vi "ExportDialog.vi"(0 "Int duplex ctl":refnum<vi>, 1 "16 bit ctl":refnum<vi>, 2 "coincidence image ctl":refnum<vi>, 3 "Path":refnum<vi>, 4 "notes 2":refnum<vi>) -> ()   [LabVIEW 2009]
uses:
  <vilib>/vision/Image Controls.llb/IMAQ Image.ctl
panel:
  in  "I16-File":bool
  in  "16 bit Image":bool
  in  "colorpal 16bit":T1(ring)
  in  "stop":bool
  in  "coincidence":bool
  in  "Int dup":bool
  in  "RGB/False":bool
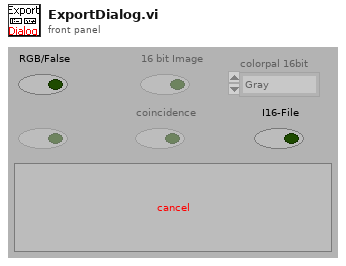
[diagram p1: front panel]
types:
  T1 = enum32{"Gray", "Binary", "Gradient", "Rainbow", "Temperature"}
  T2 = enum16{"Ini", "Get", "Set", "Refresh", "dump", "move", "name"}
  T3 = enum16{"Ini", "Dump", "Colorpal", "Input", "Get"}
  T4 = typedef "IMAQ Image.ctl" = refnum<image>
  T5 = enum16{"Get", "Set", "Change", "ini", "clear", "draw", "draw false"}
  T6 = enum16{"Ini", "Get", "Set", "Draw", "Colorpal", "Dump"}
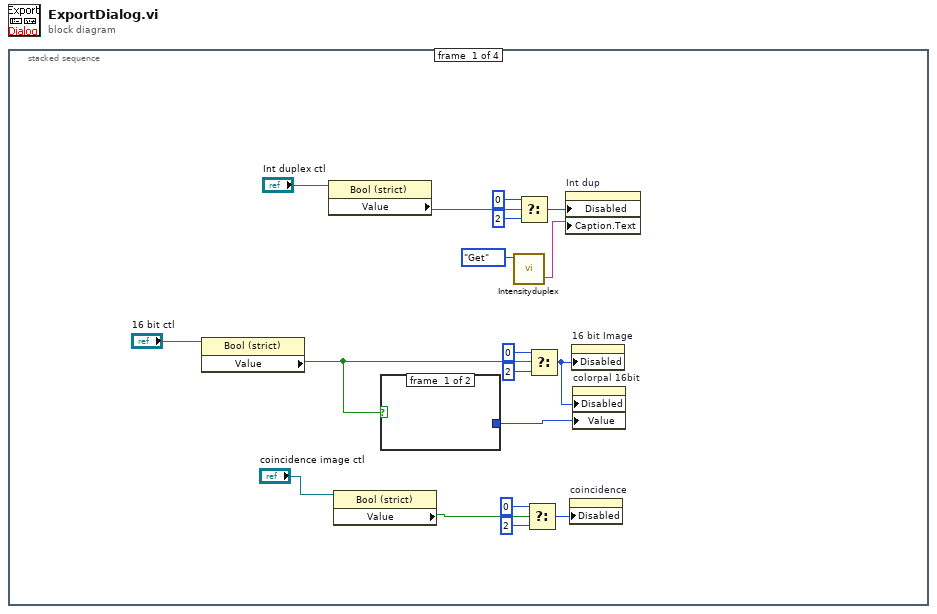
[diagram p0: block diagram]
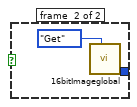
[diagram p2: hidden frame]
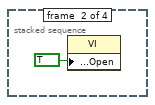
[diagram p3: hidden frame]
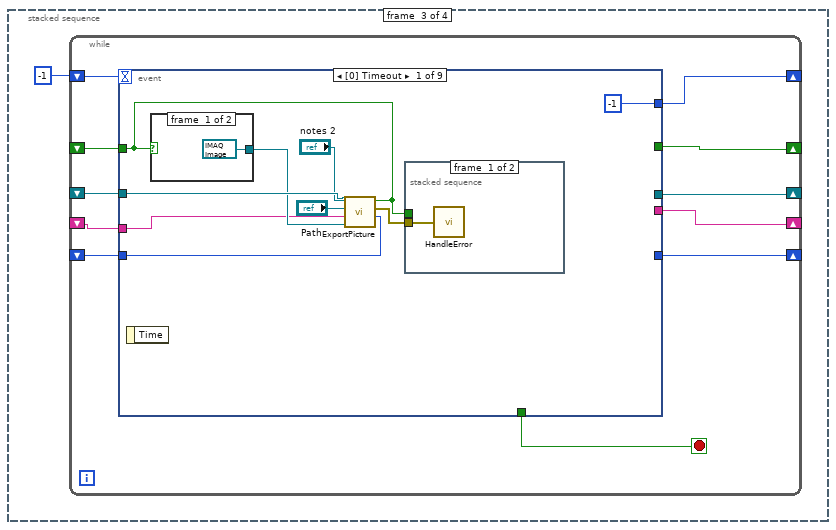
[diagram p4: hidden frame]
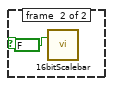
[diagram p6: hidden frame]
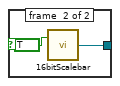
[diagram p7: hidden frame]
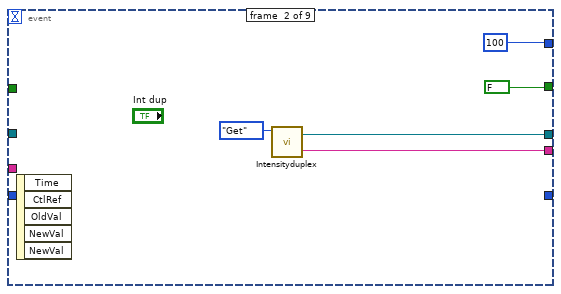
[diagram p8: hidden frame]
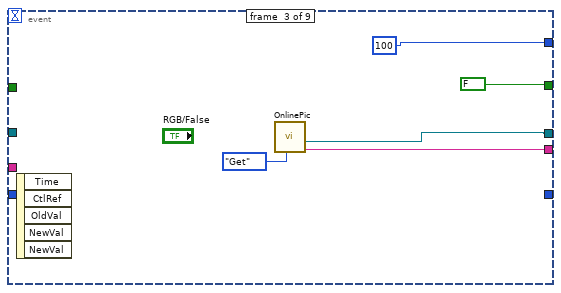
[diagram p9: hidden frame]
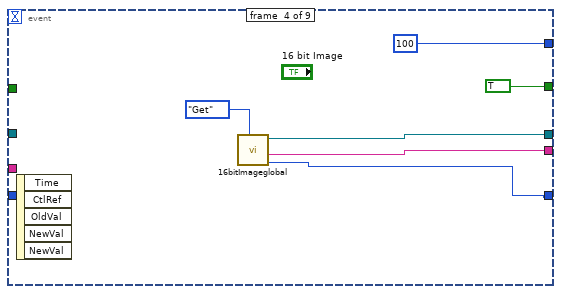
[diagram p10: hidden frame]
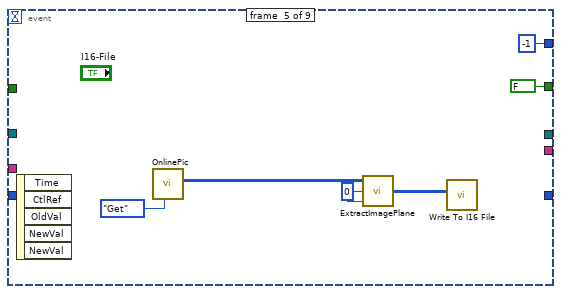
[diagram p11: hidden frame]
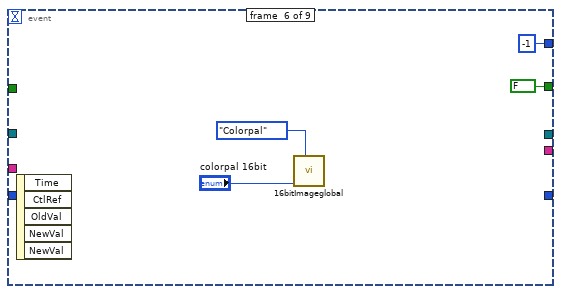
[diagram p12: hidden frame]
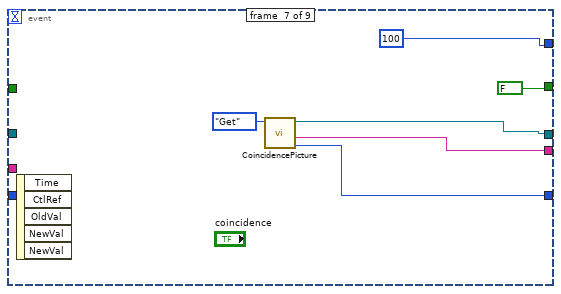
[diagram p13: hidden frame]
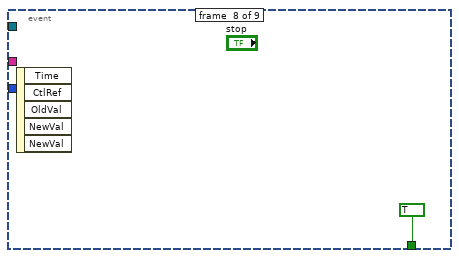
[diagram p14: hidden frame]
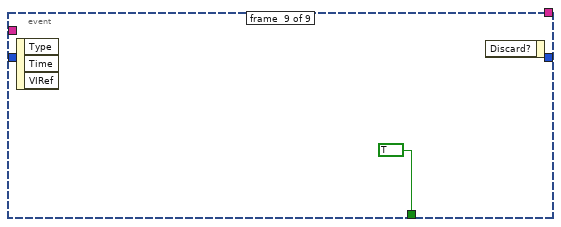
[diagram p15: hidden frame]
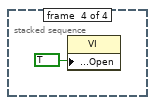
[diagram p16: hidden frame]
diagram:
  n1 = stacked-sequence {
    frame #0 {
      n2 = property on="Property Node" class="Bool (strict)"(reference="16 bit ctl") -> ("Value"=w2:bool)  [unwired: 1 in, 2 out]
      n3 = property on="Property Node" class="Bool (strict)"(reference="Int duplex ctl") -> ("Value"=w13:bool)  [unwired: 1 in, 2 out]
      n4 = property on="Property Node" class="Bool (strict)"(reference="coincidence image ctl") -> ("Value"=w9:bool)  [unwired: 1 in, 2 out]
      n5 = case shown="False" w2 {
        tunnel: [_ w19] -> w3
        frame #0 {
        }
        frame #1 {
          n6 = call "16bitImageglobal.vi"("Enum"=T3."Get") -> ("Palette Number (gray) 2"=w19:T1)  [unwired: 4 in, 3 out]
        }
      }
      n7 = call "Intensityduplex.vi"("Enum"=T2."Get") -> ("title out"=w10:string)  [unwired: 4 in, 1 out]
      n8 = Select(t=0, s=w13, f=2) -> (s? t:f=w14:i32)
      n9 = Select(t=0, s=w9, f=2) -> (s? t:f=w6:i32)
      n10 = Select(t=0, s=w2, f=2) -> (s? t:f=w4:i32)
      n11 = property on="Int dup" class="Bool"("Disabled"=w14, "Caption.Text"=w10) -> ()  [unwired: 2 in, 2 out]
      n12 = property on="coincidence" class="Bool"("Disabled"=w6) -> ()  [unwired: 2 in, 2 out]
      n13 = property on="16 bit Image" class="Bool"("Disabled"=w4) -> ()  [unwired: 2 in, 2 out]
      n14 = property on="colorpal 16bit" class="Enum (strict)"("Disabled"=w4, "Value"=w3) -> ()  [unwired: 2 in, 2 out]
    }
    frame #1 {
      n15 = property class="VI"("Front Panel Window:Open"=TRUE) -> ()  [unwired: 2 in, 2 out]
    }
    frame #2 {
      n16 = while {
        shift-right: [w31] -> _
        shift-left: -1 -> [w32]
        shift-right: [w30] -> _
        shift-left: _ -> [w25]
        shift-right: [w29] -> _
        shift-left: _ -> [w26]
        shift-right: [w28] -> _
        shift-left: _ -> [w27]
        shift-right: [w24] -> _
        shift-left: _ -> [w23]
        stop <- w33 stop-if-true
        n17 = event shown="[0] Timeout" {
          selector: _ -> [_ _ _ _ _ _ _ _ _]
          dyn-events: _ -> [_ _ _ _ _ _ _ _ _]
          timeout: w32 -> [_ _ _ _ _ _ _ _ _]
          tunnel: [_ _ _ _ _ _ _ TRUE TRUE] -> w33
          tunnel: [-1 100 100 100 -1 -1 100 _ _] -> w31
          tunnel: [_ w51 w56 w61 _ _ w77 _ _] -> w30
          tunnel: [_ w50 w55 w62 _ _ w78 _ _] -> w29
          tunnel: [_ FALSE FALSE TRUE FALSE FALSE FALSE _ _] -> w28
          tunnel: w27 -> [w34 _ _ _ _ _ _ _ _]
          tunnel: w26 -> [w36 _ _ _ _ _ _ _ _]
          tunnel: w25 -> [w39 _ _ _ _ _ _ _ _]
          tunnel: [_ _ _ w59 _ _ w79 _ _] -> w24
          tunnel: w23 -> [w38 _ _ _ _ _ _ _ _]
          event #0 {
            n18 = event-data() -> ()  [unwired: 1 in, 1 out]
            n19 = case shown="True" w34 {
              tunnel: [T4 refnum ("Image Out") w47] -> w37
              frame #0 {
              }
              frame #1 {
                n20 = call "16bitScalebar.vi"("Boolean"=TRUE) -> ("Image Out"=w47:T4)  [unwired: 1 in]
              }
            }
            n21 = call "ExportPicture.vi"("Palette Number (gray)"=w38, "16bit Image?"=w34, "Image"=w39, "Image Scalebar"=w37, "name input"=w36, "Path"="Path", "notes 2"="notes 2") -> ("error out"=w41:errorcluster)  [unwired: 1 out]
            n22 = stacked-sequence {
              tunnel: w41 -> [w43 _]
              tunnel: w34 -> [_ w44]
              frame #0 {
                n23 = call "HandleError.vi"("error in (no error)"=w43) -> ()
              }
              frame #1 {
                n24 = case shown="True" w44 {
                  frame #0 {
                  }
                  frame #1 {
                    n25 = call "16bitScalebar.vi"("Boolean"=FALSE) -> ()  [unwired: 1 in, 1 out]
                  }
                }
              }
            }
          }
          event #1 {
            n26 = event-data() -> ()  [unwired: 1 in, 5 out]
            n27 = call "Intensityduplex.vi"("Enum"=enum16{"Ini", "Get", "Set", "Refresh", "dump"}."Get") -> ("Image Duplicate (out)"=w51:T4, "title out"=w50:string)  [unwired: 4 in]
          }
          event #2 {
            n28 = event-data() -> ()  [unwired: 1 in, 5 out]
            n29 = call "OnlinePic.vi"("action"=enum16{"Get", "Set", "Change", "ini"}."Get" ("Enum")) -> ("Title"=w55:string, "Image Out (duplicate)"=w56:T4)  [unwired: 6 in, 3 out]
          }
          event #3 {
            n30 = event-data() -> ()  [unwired: 1 in, 5 out]
            n31 = call "16bitImageglobal.vi"("Enum"=T3."Get") -> ("Palette Number (gray) 2"=w59:T1, "Title"=w62:string, "Image Out (duplicate)"=w61:T4)  [unwired: 4 in, 1 out]
          }
          event #4 {
            w69 = u32 0 ("Plane")
            n32 = event-data() -> ()  [unwired: 1 in, 5 out]
            n33 = call "OnlinePic.vi"("action"=T5."Get" ("Enum")) -> ("Sum of Photons"=w67:u32[][][][])  [unwired: 6 in, 4 out]
            n34 = call "ExtractImagePlane.vi"("Router"=w69, "Plane"=w69, "Trace"=w67) -> ("Intensity"=w66:u32[][])
            n35 = call "Write To I16 File.vi"("2D array"=w66) -> ()  [unwired: 6 in, 1 out]
          }
          event #5 {
            n36 = event-data() -> ()  [unwired: 1 in, 5 out]
            n37 = call "16bitImageglobal.vi"("Enum"=T3."Colorpal", "Palette Number (gray)"="colorpal 16bit") -> ()  [unwired: 3 in, 4 out]
          }
          event #6 {
            n38 = event-data() -> ()  [unwired: 1 in, 5 out]
            n39 = call "CoincidencePicture.vi"("Enum"=T6."Get") -> ("Palette Number (gray) 2"=w79:T1, "String"=w78:string, "Image Out"=w77:T4)  [unwired: 6 in]
          }
          event #7 {
            n40 = event-data() -> ()  [unwired: 1 in, 5 out]
          }
          event #8 {
            n41 = event-data() -> ()  [unwired: 1 in, 3 out]
            n42 = event-data() -> ()  [unwired: 2 in, 1 out]
          }
        }
      }
    }
    frame #3 {
      n43 = property class="VI"("Front Panel Window:Open"=TRUE) -> ()  [unwired: 2 in, 2 out]
    }
  }
